vi "MonitoringPanel.vi"() -> ()   [LabVIEW 2018]
panel:
  in  "Stop":bool
  out "Low":bool
  in  "Frequency":dbl(knob) scale=5.0..20.0
  out "Photovoltaic":dbl(knob) scale=0.0..10.0
  out "Battery Level":dbl(slide) scale=0.0..10.0
  out "Diesel Chart":dynamicdata(graph)
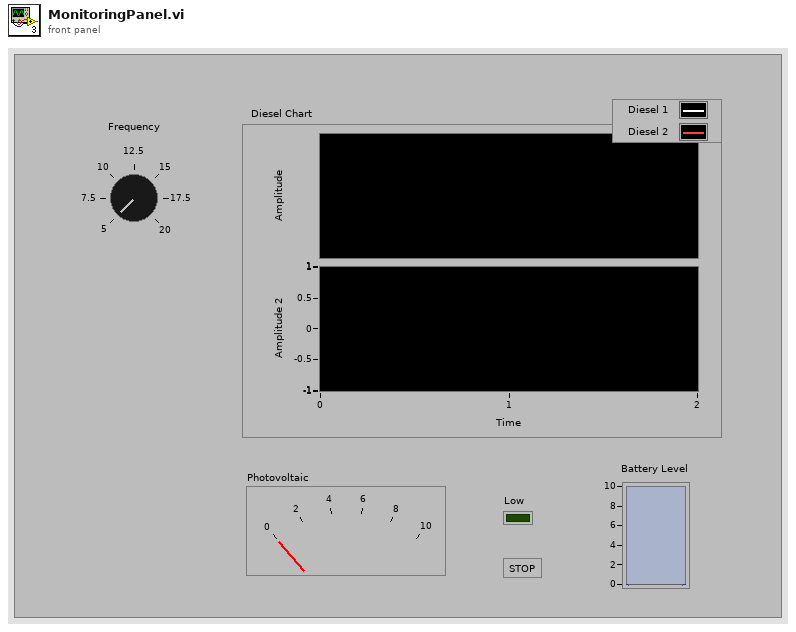
[diagram p1: front panel]
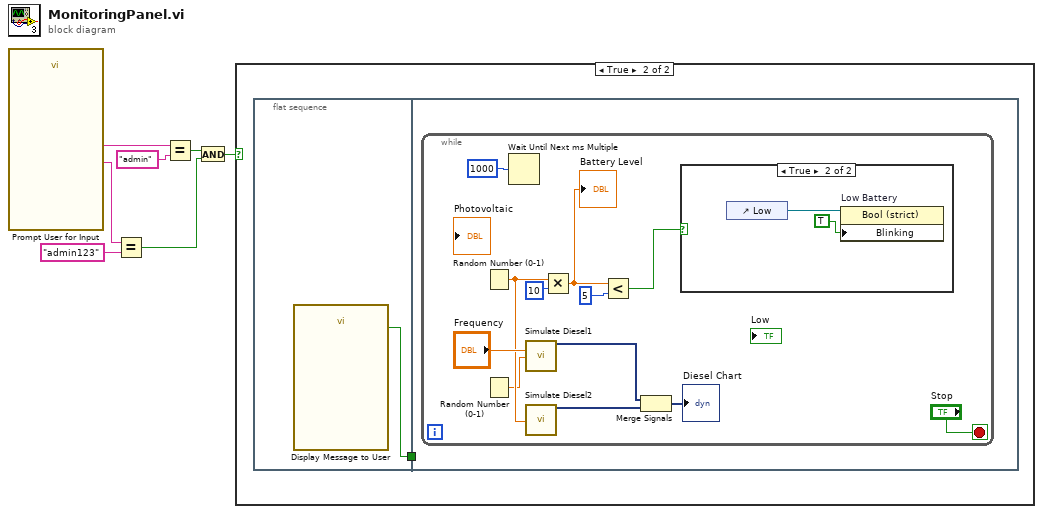
[diagram p0: block diagram]
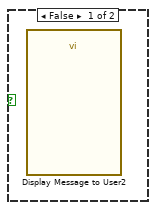
[diagram p2: hidden frame]
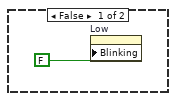
[diagram p3: hidden frame]
diagram:
  n1 = call "Prompt User for Input"() -> ("Password"=w6:string, "User"=w7:string)  [unwired: 16 in, 2 out]
  n2 = Equal?(x=w6, y="admin123") -> (x = y?=w4:bool)
  n3 = Equal?(x=w7, y="admin") -> (x = y?=w5:bool)
  n4 = And(x=w5, y=w4) -> (x .and. y?=w1:bool)
  n5 = case shown="True" w1 {
    frame False {
      n6 = call "Display Message to User2"() -> ()  [unwired: 10 in, 2 out]
    }
    frame True {
      n7 = flat-sequence {
        tunnel: [w9] -> w8
        tunnel: w8 -> [_]
        frame #0 {
          n8 = call "Display Message to User"() -> ("OK"=w9:bool)  [unwired: 10 in, 1 out]
        }
        frame #1 {
          n9 = while {
            stop <- "Stop" stop-if-true
            n10 = Random Number (0-1)() -> (number: 0 to 1=w17:dbl)
            n11 = Random Number (0-1)() -> (number: 0 to 1=w13:dbl)
            n12 = Wait Until Next ms Multiple(millisecond multiple=1000) -> ()  [unwired: 1 out]
            n13 = call "Simulate Diesel1"("Frequency"="Frequency", "Amplitude"=w13) -> ("Sine"=w14:dynamicdata)  [unwired: 12 in, 1 out]
            n14 = call "Simulate Diesel2"("Amplitude"=w17) -> ("Triangle"=w16:dynamicdata)  [unwired: 13 in, 1 out]
            n15 = Multiply(x=w17, y=10) -> (x*y=w19:dbl)
            "Battery Level" <- w19
            n16 = Less?(x=w19, y=5) -> (x < y?=w20:bool)
            n17 = Merge Signals(w14, w16) -> (→"Diesel Chart":dynamicdata)
            n18 = case shown="True" w20 {
              frame False {
                n19 = property on="Low" class="Bool (strict)"("Blinking"=FALSE) -> ()  [unwired: 2 in, 2 out]
              }
              frame True {
                n20 = control-ref of="Low"() -> (w24:refnum<vi>)
                n21 = property on="Low Battery" class="Bool (strict)"(reference=w24, "Blinking"=TRUE) -> ()  [unwired: 1 in, 2 out]
              }
            }
          }
        }
      }
    }
  }
